vi "Agilent 3458 Acquire Sub-Sampling Measurement.vi"() -> ()   [LabVIEW 2010]
doc: "Configures and Reads measurements using the sub-sampling method. This VI shows precisely how to configure and use sub-sampling. Note that this VI uses level triggering as the source for the sub-sampling."
uses:
  <instrlib>/Agilent 3458/Public/Data/Read Measurement(Multiple Points).vi
  <instrlib>/Agilent 3458/Agilent 3458.lvlib
panel:
  in  "Manual Range (1.00)":dbl=1.0 format="%_3g"
  out "Measurements":sgl[](array[numeric])
  in  "Manual Resolution (2: 6.5 digits)":enum16{"4.5", "5.5", "6.5", "7.5", "8.5"}(ring)=enum."6.5"
  in  "Percentage (0%)":dbl
  in  "Slope (1:Positive)":u16(ring)=1 items=["Negative", "Positive"]
  in  "Coupling (0:AC)":u16(ring) items=["AC", "DC"]
  in  "Function(0:Sub-Sampling DC)":u16(ring) items=["Sub-Sampling DC", "Sub-Sampling AC"]
  in  "Maximum Time (10000 ms)":u32=10000
  in  "Sample Interval (20E-6 s)":dbl=2e-05 format="%#.6g"
  in  "Sample Count (1024)":dbl=1024.0 format="%#.6g"
  in  "VISA resource name":refnum<visa-resource-name>
  # "(c) 2007  National Instruments.  ALL RIGHTS RESERVED."
  # "Level Triggering"
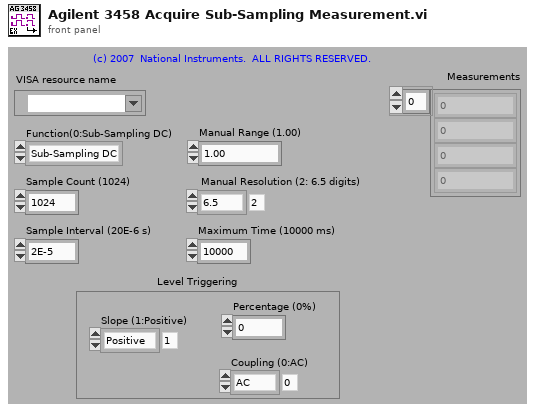
[diagram p1: front panel]
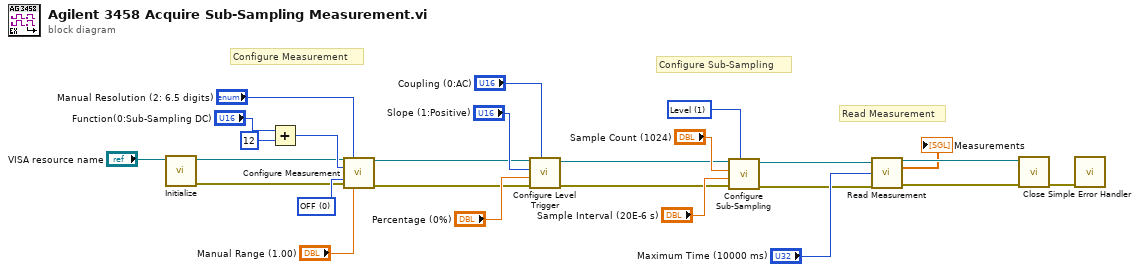
[diagram p0: block diagram]
diagram:
  w17 = u16 1 items=["External", "Level"] ("Sub-Sampling Source(1:Level)")
  w25 = u16 0 items=["OFF", "ON", "ONCE"] ("Auto Range (1:ON)")
  # "Configure Measurement"
  # "Configure Sub-Sampling"
  # "Read Measurement"
  n1 = call <instrlib>:"Initialize.vi"("VISA resource name"="VISA resource name") -> ("error out"=w6:errorcluster, "VISA resource name out"=w7:refnum<visa-resource-name>)  [unwired: 9 in]
  n2 = Add(x="Function(0:Sub-Sampling DC)", y=u16 12) -> (x+y=w18:u16)
  n3 = call <instrlib>:"Configure Measurement.vi"("VISA resource name"=w7, "Manual Resolution (2: 6.5 digits)"="Manual Resolution (2: 6.5 digits)", "Function (0: DC Voltage)"=w18, "Auto Range (1:ON)"=w25, "error in (no error)"=w6, "Manual Range (1.00)"="Manual Range (1.00)") -> ("VISA resource name out"=w11:refnum<visa-resource-name>, "error out"=w10:errorcluster)  [unwired: 8 in]
  n4 = call <instrlib>:"Configure Level Trigger.vi"("Coupling (0:AC)"="Coupling (0:AC)", "error in (no error)"=w10, "Percentage (0%)"="Percentage (0%)", "Slope (1:Positive)"="Slope (1:Positive)", "VISA resource name"=w11) -> ("error out"=w8:errorcluster, "VISA resource name out"=w9:refnum<visa-resource-name>)  [unwired: 5 in]
  n5 = call <instrlib>:"Configure Sub-Sampling.vi"("Sub-Sampling Source(1:Level)"=w17, "error in (no error)"=w8, "Sample Interval (20E-6 s)"="Sample Interval (20E-6 s)", "Sample Count (1024)"="Sample Count (1024)", "VISA resource name"=w9) -> ("error out"=w15:errorcluster, "VISA resource name out"=w16:refnum<visa-resource-name>)  [unwired: 5 in]
  n6 = call-poly <instrlib>:"Read Measurement.vi"("VISA resource name"=w16, "Maximum Time (10000 ms)"="Maximum Time (10000 ms)", "error in (no error)"=w15) -> ("VISA resource name out"=w5:refnum<visa-resource-name>, "Measurements"=→"Measurements":sgl[], "error out"=w4:errorcluster)  [unwired: 10 in]
  n7 = call <instrlib>:"Close.vi"("error in (no error)"=w4, "VISA resource name"=w5) -> ("error out"=w21:errorcluster)  [unwired: 9 in]
  n8 = call <vilib>:"Simple Error Handler.vi"("error in (no error)"=w21) -> ()  [unwired: 4 in, 5 out]
